vi "Close.vi"(8 "error in (no error)":errorcluster, 11 "ByteGSWebAPI-V0 in":refnum<class "ByteGSWebAPI-V0.lvclass">) -> (0 "error out":errorcluster, 3 "ByteGSWebAPI-V0 out":refnum<class "ByteGSWebAPI-V0.lvclass">)   [LabVIEW 2019, in "ByteGSWebAPI.lvlib" / "ByteGSWebAPI-V0.lvclass"]
uses:
  ByteGSWebAPI-V0.lvclass
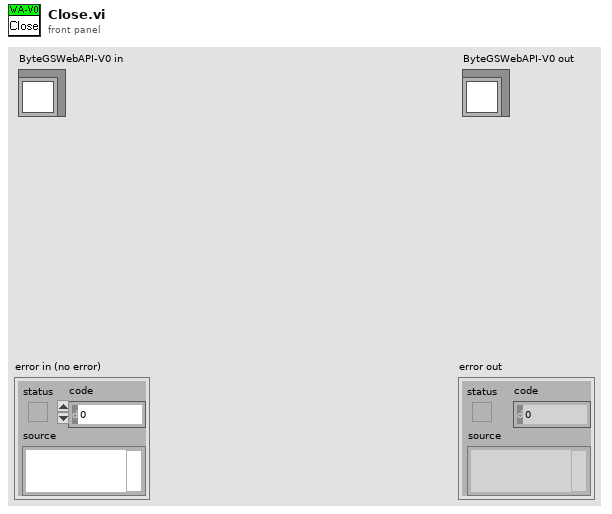
[diagram p1: front panel]
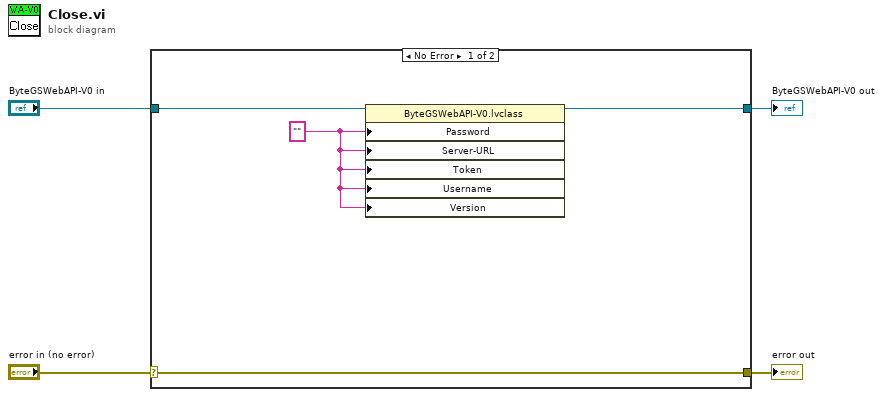
[diagram p0: block diagram]
diagram:
  n1 = case shown="No Error" "error in (no error)" {
    selector: "error in (no error)" -> [w8 w10]
    tunnel: [w8 w10] -> w3
    tunnel: [w7 w9] -> w1
    tunnel: "ByteGSWebAPI-V0 in" -> [w6 w9]
    frame No Error {
      w5 = "" ("Password")
      n2 = property class="ByteGSWebAPI-V0.lvclass"(reference=w6, "Password"=w5, "Server-URL"=w5, "Token"=w5, "Username"=w5, "Version"=w5) -> (reference out=w7:refnum<class "ByteGSWebAPI-V0.lvclass">)  [unwired: 1 in, 1 out]
    }
    frame Error {
    }
  }
  "error out" <- w3
  "ByteGSWebAPI-V0 out" <- w1
